vi "GlobalDAQ.vi"() -> ()   [LabVIEW 2011]
uses:
  C:/Program Files (x86)/National Instruments/LabVIEW 2011/vi.lib/ULx/ULx_LV.dll
  Program Files (x86)/National Instruments/LabVIEW 2011/vi.lib/ULx/ULx_LV.dll
panel:
  out "semaphore":T1
  out "DAQ task out":refnum<k24>
  in  "Fly Detection":T2
  out "DAQ error":errorcluster
  out "DAQ task":refnum<k24>
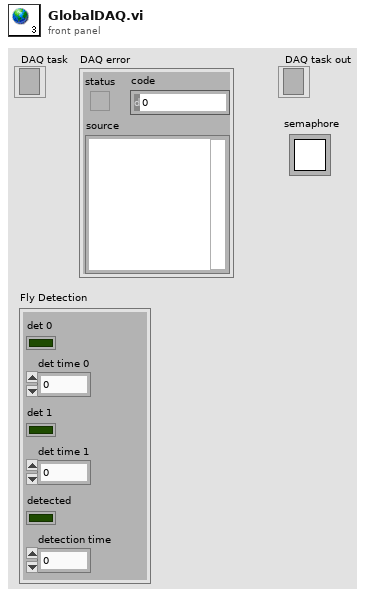
[diagram p1: front panel]
types:
  T1 = typedef "Semaphore RefNum" = refnum<k1>
  T2 = cluster{"det 0":bool, "det time 0":u32, "det 1":bool, "det time 1":u32, "detected":bool, "detection time":u32}
diagram:
